vi "arb_rotation_matrix.vi"(1 "Unit Vector":cluster{dbl, dbl, dbl}, 2 "theta":dbl) -> (0 "Real Matrix":T1)   [LabVIEW 2015]
uses:
  <vilib>/Analysis/Matrix/Datatypes/RealMatrix.ctl
  <vilib>/Analysis/Matrix/Numeric/Conversions/Array To Matrix - RA2.vi
  <vilib>/Analysis/Matrix/NI_Matrix.lvlib
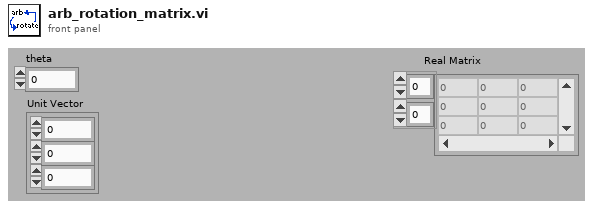
[diagram p1: front panel]
types:
  T1 = typedef "NI_Matrix.lvlib/RealMatrix.ctl" = dbl[][]
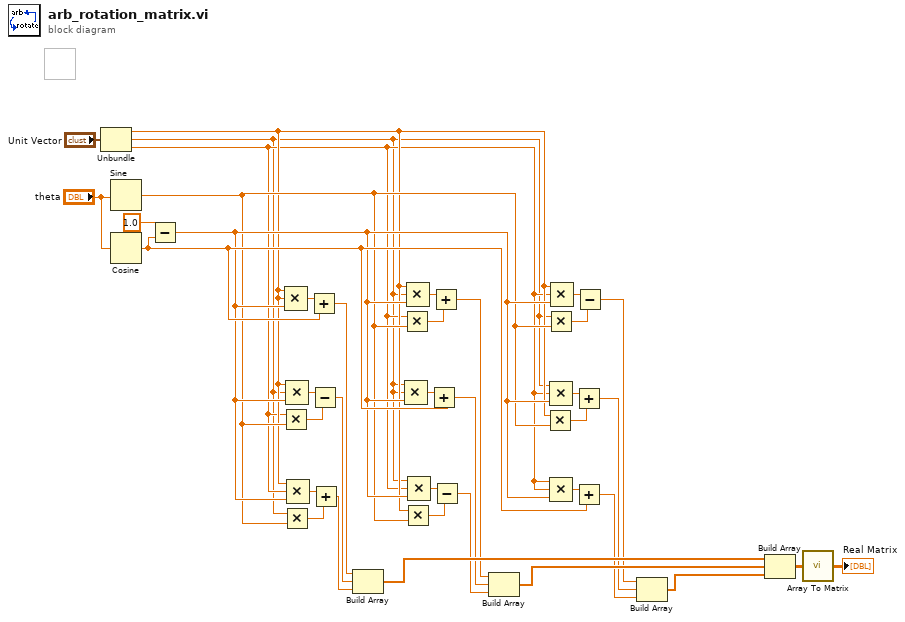
[diagram p0: block diagram]
diagram:
  n1 = Unbundle("Unit Vector") -> (w3:dbl, w1:dbl, w2:dbl)
  n2 = Sine(x="theta") -> (sin(x)=w18:dbl)
  n3 = Cosine(x="theta") -> (cos(x)=w20:dbl)
  n4 = Subtract(x=1.0, y=w20) -> (x-y=w19:dbl)
  n5 = Multiply(x=w2, y=w18) -> (x*y=w29:dbl)
  n6 = Multiply(x=w1, y=w18) -> (x*y=w24:dbl)
  n7 = Compound Arithmetic op=MULTIPLY(w3, w3, w19) -> (w37:dbl)
  n8 = Compound Arithmetic op=MULTIPLY(w3, w1, w19) -> (w30:dbl)
  n9 = Compound Arithmetic op=MULTIPLY(w3, w2, w19) -> (w25:dbl)
  n10 = Add(x=w37, y=w20) -> (x+y=w17:dbl)
  n11 = Subtract(x=w30, y=w29) -> (x-y=w16:dbl)
  n12 = Add(x=w25, y=w24) -> (x+y=w15:dbl)
  n13 = Build Array(w17, w16, w15) -> (w14:dbl[])
  n14 = Multiply(x=w2, y=w18) -> (x*y=w33:dbl)
  n15 = Multiply(x=w3, y=w18) -> (x*y=w22:dbl)
  n16 = Compound Arithmetic op=MULTIPLY(w1, w1, w19) -> (w28:dbl)
  n17 = Compound Arithmetic op=MULTIPLY(w3, w1, w19) -> (w34:dbl)
  n18 = Compound Arithmetic op=MULTIPLY(w1, w2, w19) -> (w23:dbl)
  n19 = Add(x=w28, y=w20) -> (x+y=w12:dbl)
  n20 = Add(x=w34, y=w33) -> (x+y=w13:dbl)
  n21 = Subtract(x=w23, y=w22) -> (x-y=w11:dbl)
  n22 = Build Array(w13, w12, w11) -> (w10:dbl[])
  n23 = Multiply(x=w3, y=w18) -> (x*y=w26:dbl)
  n24 = Multiply(x=w1, y=w18) -> (x*y=w31:dbl)
  n25 = Compound Arithmetic op=MULTIPLY(w1, w2, w19) -> (w27:dbl)
  n26 = Compound Arithmetic op=MULTIPLY(w2, w2, w19) -> (w21:dbl)
  n27 = Compound Arithmetic op=MULTIPLY(w3, w2, w19) -> (w32:dbl)
  n28 = Add(x=w27, y=w26) -> (x+y=w8:dbl)
  n29 = Add(x=w21, y=w20) -> (x+y=w7:dbl)
  n30 = Subtract(x=w32, y=w31) -> (x-y=w9:dbl)
  n31 = Build Array(w9, w8, w7) -> (w6:dbl[])
  n32 = Build Array(w14, w10, w6) -> (w5:dbl[][])
  n33 = call-poly <vilib>:"Array To Matrix.vi"("Real 2D Array"=w5) -> ("Real Matrix"=→"Real Matrix":T1)
